vi "attribute_read_int32_simple.vi"(5 "Repeated Capability":string, 7 "Attribute":T1={"Identifier"="", "Descriptive Name"="", "Data Type"=enum."Integer 32", "Command"="", "Access"=enum."Read/Write", "Range Table"="", "Read Callback"="", "Write Callback"="", "Supported Models"="", "Instrument Options"="", "Index"=0, "OPC Wait"=FALSE, "No Status Check"=FALSE, "Cache Only"=FALSE}, 8 "error in":errorcluster caption="error in (no error)", 10 "Direct Attribute ID (\"\")":string, 11 "VISA resource name":refnum<visa-resource-name>) -> (0 "error out":errorcluster, 2 "Int32 out":i32, 3 "VISA resource name out":refnum<visa-resource-name>)   [LabVIEW 2020, in "Rohde&Schwarz RTx Oscilloscopes.lvlib" / "rsidr_core.lvlib"]
uses:
  rsidr_core.lvlib
  type_Attribute.ctl
  type_Attribute_Data_Type.ctl
  type_ReadWriteAccess.ctl
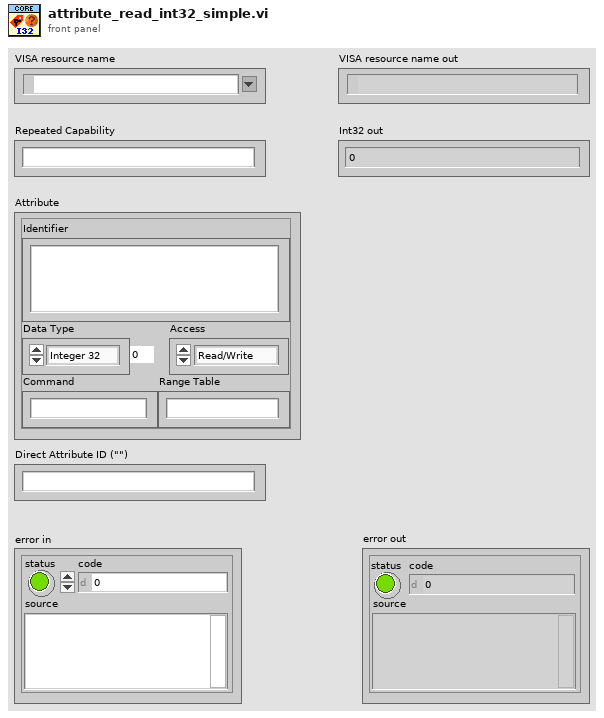
[diagram p1: front panel]
types:
  T1 = typedef "Rohde&Schwarz RTx Oscilloscopes.lvlib/rsidr_core.lvlib/type_Attribute.ctl" = cluster{"Identifier":string, "Descriptive Name":string, "Data Type":T2, "Command":string, "Access":T3, "Range Table":string, "Read Callback":string, "Write Callback":string, "Supported Models":string, "Instrument Options":string, "Index":i32, "OPC Wait":bool, "No Status Check":bool, "Cache Only":bool}
  T2 = typedef "Rohde&Schwarz RTx Oscilloscopes.lvlib/rsidr_core.lvlib/type_Attribute_Data_Type.ctl" = enum16{"Integer 32", "Double", "String", "Boolean", "None", "Integer 64", "RawString"}
  T3 = typedef "Rohde&Schwarz RTx Oscilloscopes.lvlib/rsidr_core.lvlib/type_ReadWriteAccess.ctl" = enum16{"Read Only", "Write Only", "Read/Write"}
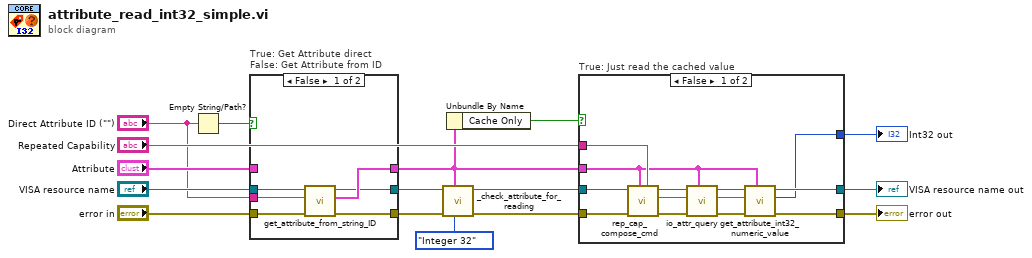
[diagram p0: block diagram]
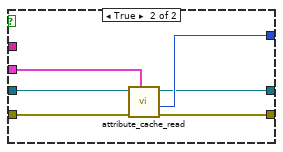
[diagram p3: hidden frame]
diagram:
  n1 = Empty String/Path?(string/path="Direct Attribute ID (\"\")") -> (empty?=w2:bool)
  n2 = case "True: Get Attribute direct\nFalse: Get Attribute from ID" shown="False" w2 {
    tunnel: "error in" -> [w20 w24]
    tunnel: [w18 w24] -> w7
    tunnel: "Direct Attribute ID (\"\")" -> [w22 _]
    tunnel: "Attribute" -> [_ w25]
    tunnel: [w21 w25] -> w3
    tunnel: "VISA resource name" -> [w19 w23]
    tunnel: [w17 w23] -> w6
    frame False {
      n3 = call "get_attribute_from_string_ID.vi"("error in"=w20, "Attribute ID in"=w22, "VISA resource name"=w19) -> ("error out"=w18:errorcluster, "Attribute out"=w21:T1, "VISA resource name out"=w17:refnum<visa-resource-name>)  [unwired: 6 in]
    }
    frame True {
    }
  }
  n4 = call "_check_attribute_for_reading.vi"("Expected Data Type"=type_Attribute_Data_Type."Integer 32", "Attribute"=w3, "error in"=w7, "VISA resource name"=w6) -> ("error out"=w11:errorcluster, "VISA resource name out"=w10:refnum<visa-resource-name>)  [unwired: 6 in]
  n5 = Unbundle By Name(w3) -> ("Cache Only"=w1:bool)
  n6 = case "True: Just read the cached value" shown="False" w1 {
    tunnel: "Repeated Capability" -> [w38 _]
    tunnel: [w37 w40] -> w14
    tunnel: [w36 w39] -> w13
    tunnel: [w35 w41] -> w15
    tunnel: w10 -> [w34 w43]
    tunnel: w11 -> [w33 w44]
    tunnel: w3 -> [w26 w42]
    frame False {
      n7 = call "rep_cap_compose_cmd.vi"("Repeated Capability"=w38, "Attribute"=w26, "error in"=w33, "VISA resource name"=w34) -> ("error out"=w32:errorcluster, "Command out"=w31:string, "VISA resource name out"=w30:refnum<visa-resource-name>)  [unwired: 5 in]
      n8 = call "io_attr_query.vi"("Attribute"=w26, "error in"=w32, "write buffer"=w31, "VISA resource name"=w30) -> ("error out"=w29:errorcluster, "read buffer"=w27:string, "VISA resource name out"=w28:refnum<visa-resource-name>)  [unwired: 5 in]
      n9 = call "get_attribute_int32_numeric_value.vi"("Attribute"=w26, "error in"=w29, "Cmd Value in"=w27, "VISA resource name"=w28) -> ("error out"=w37:errorcluster, "Int32 value out"=w35:i32, "VISA resource name out"=w36:refnum<visa-resource-name>)  [unwired: 5 in]
    }
    frame True {
      n10 = call "attribute_cache_read.vi"("Attribute"=w42, "error in"=w44, "VISA resource name"=w43) -> ("error out"=w40:errorcluster, "Int32 out"=w41:i32, "VISA resource name out"=w39:refnum<visa-resource-name>)  [unwired: 1 in, 5 out]
    }
  }
  "error out" <- w14
  "VISA resource name out" <- w13
  "Int32 out" <- w15
